vi "Is_Channel_Vaild.vi"(1 "输入数组":string[](array[string])) -> (0 "元素不重复？（真：不重复，假：有重复元素）":bool)   [LabVIEW 2024]
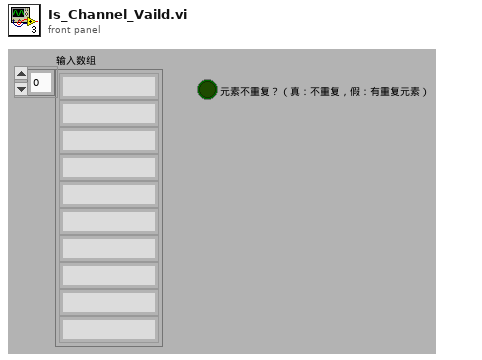
[diagram p1: front panel]
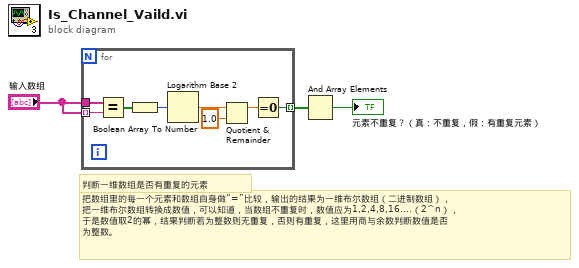
[diagram p0: block diagram]
diagram:
  # "把数组里的每一个元素和数组自身做“=”比较，输出的结果为一维布尔数组（二进制数组），\n把一维布尔数组转换成数值，可以知道，当数组不重复时，数值应为1,2,4,8,16....（2^n），\n于是数值取2的幂，结果判断若为整数则无重复，否则有重复，这里用商与余数判断数值是否\n为整数。"
  # "判断一维数组是否有重复的元素"
  n1 = for {
    tunnel: "输入数组" -> [w6] mode=indexing
    tunnel: "输入数组" -> [w5]
    tunnel: [w4] -> w3 mode=indexing
    n2 = Equal?(x=w5, y=w6) -> (x = y?=w7:bool[])
    n3 = Boolean Array To Number(Boolean array=w7) -> (number=w8:u32)
    n4 = Logarithm Base 2(1:w8) -> (0:w9:dbl)
    n5 = Quotient & Remainder(x=w9, y=1.0) -> (x-y*floor(x/y)=w11:dbl)  [unwired: 1 out]
    n6 = Equal To 0?(x=w11) -> (x = 0?=w4:bool)
  }
  n7 = And Array Elements(Boolean array=w3) -> (logical AND=→"元素不重复？（真：不重复，假：有重复元素）":bool)
